vi "Set Friendships.vi"(10 "Manifest Ancestor":refnum<vi>, 11 "Class Ref Map":variant) -> (3 "Class Ref Map Dup":variant)   [LabVIEW 2013]
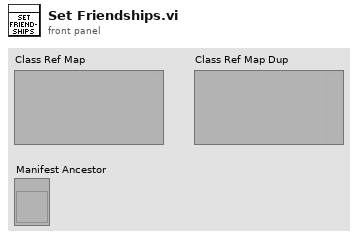
[diagram p1: front panel]
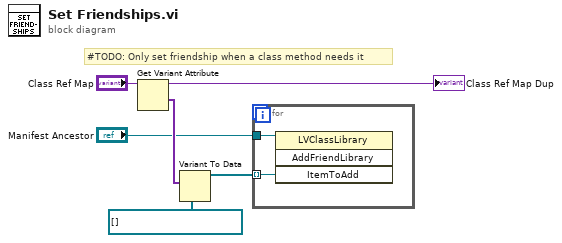
[diagram p0: block diagram]
diagram:
  # "#TODO: Only set friendship when a class method needs it"
  n1 = Get Variant Attribute(Variant="Class Ref Map") -> (duplicate Variant=→"Class Ref Map Dup":variant, values=w4:variant[])  [unwired: 3 in, 2 out]
  n2 = Variant To Data(type=refnum<vi>[] [], Variant=w4) -> (data=w2:refnum<vi>[])  [unwired: 1 in, 1 out]
  n3 = for {
    tunnel: w2 -> [w7] mode=indexing
    tunnel: "Manifest Ancestor" -> [w8]
    n4 = invoke class="LVClassLibrary" method="AddFriendLibrary"(reference=w8, "ItemToAdd"=w7) -> ()  [unwired: 2 in, 4 out]
  }
